vi "eodreader_singlepass.vi"() -> ()   [LabVIEW 2013]
panel:
  out "Waveform Graph":i16[](graph)
  out "npts":i32
  out "adrange":sgl format="%.2f"
  out "samprate":u32
  out "polarity":i8
  out "nbytes":i8
  out "nbits":i32
  out "eod_text":string
  out "nchar":i32
  out "wave":i16[](array[numeric])
  out "userdata":sgl[](array[numeric]) format="%.2f"
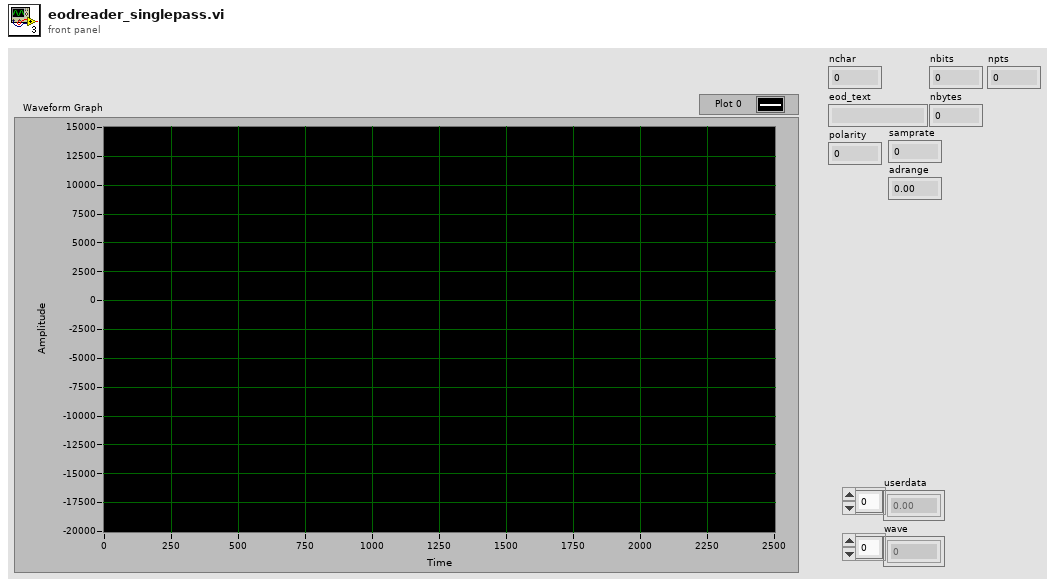
[diagram p1: front panel]
types:
  T1 = enum16{"open", "replace", "create", "open or create", "replace or create", "replace or create with confirmation"}
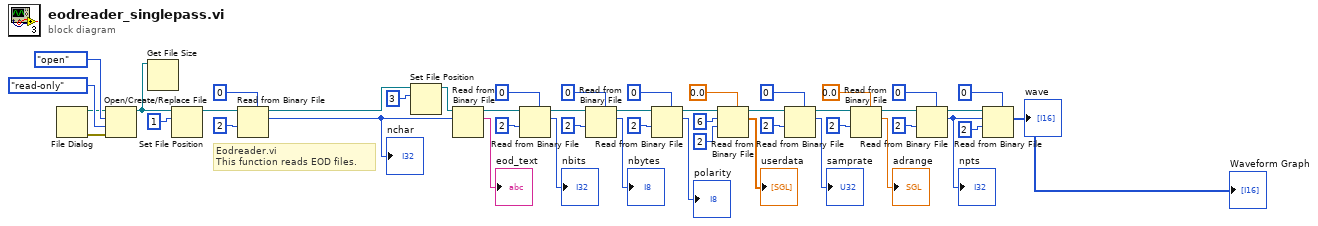
[diagram p0: block diagram]
diagram:
  # "Eodreader.vi\nThis function reads EOD files."
  n1 = File Dialog() -> (0:w44:errorcluster, 3:w45:path)  [unwired: 7 in, 2 out]
  n2 = Open/Create/Replace File(file path (use dialog)=w45, error in=w44, operation (0:open)=T1."open", access (0:read/write)=enum16{"read/write", "read-only", "write-only"}."read-only") -> (refnum out=w43:refnum<file>)  [unwired: 2 in, 2 out]
  n3 = Get File Size(file=w43) -> ()  [unwired: 1 in, 3 out]
  n4 = Set File Position(offset (in bytes) (0)=1, refnum=w43) -> (refnum out=w40:refnum<file>)  [unwired: 2 in, 1 out]
  n5 = Read from Binary File(5:u8 0, 9:2, 11:w40) -> (2:w2:u8, 3:w38:refnum<file>)  [unwired: 3 in, 2 out]
  "nchar" <- w2
  n6 = Set File Position(offset (in bytes) (0)=3, refnum=w38) -> (refnum out=w36:refnum<file>)  [unwired: 2 in, 1 out]
  n7 = Read from Binary File(10:w2, 11:w36) -> (2:→"eod_text":string, 3:w35:refnum<file>)  [unwired: 4 in, 2 out]
  n8 = Read from Binary File(5:i8 0, 9:2, 11:w35) -> (2:→"nbits":i8, 3:w11:refnum<file>)  [unwired: 3 in, 2 out]
  n9 = Read from Binary File(5:i8 0, 9:2, 11:w11) -> (2:→"nbytes":i8, 3:w12:refnum<file>)  [unwired: 3 in, 2 out]
  n10 = Read from Binary File(5:i8 0, 9:2, 11:w12) -> (2:→"polarity":i8, 3:w10:refnum<file>)  [unwired: 3 in, 2 out]
  n11 = Read from Binary File(5:sgl 0.0, 9:2, 10:6, 11:w10) -> (2:→"userdata":sgl[], 3:w32:refnum<file>)  [unwired: 2 in, 2 out]
  n12 = Read from Binary File(5:u32 0, 9:2, 11:w32) -> (2:→"samprate":u32, 3:w24:refnum<file>)  [unwired: 3 in, 2 out]
  n13 = Read from Binary File(5:sgl 0.0, 9:2, 11:w24) -> (2:→"adrange":sgl, 3:w18:refnum<file>)  [unwired: 3 in, 2 out]
  n14 = Read from Binary File(5:u32 0, 9:2, 11:w18) -> (2:w9:u32, 3:w19:refnum<file>)  [unwired: 3 in, 2 out]
  "npts" <- w9
  n15 = Read from Binary File(5:i16 0, 9:2, 10:w9, 11:w19) -> (2:→"wave" →"Waveform Graph":i16[])  [unwired: 2 in, 3 out]
